vi "Get Message Fields.vi"(8 "error in (no error)":errorcluster, 11 "Message ref in":u64) -> (0 "error out":errorcluster, 2 "Field refs":u64[](array[numeric]), 3 "Message ref out":u64)   [LabVIEW 2019, in "gRPC Scripting Tools.lvlib"]
uses:
  gRPC Scripting Tools.lvlib
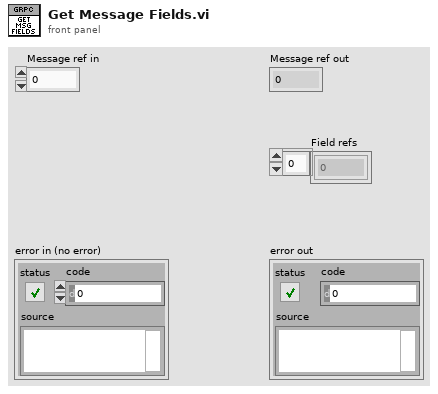
[diagram p1: front panel]
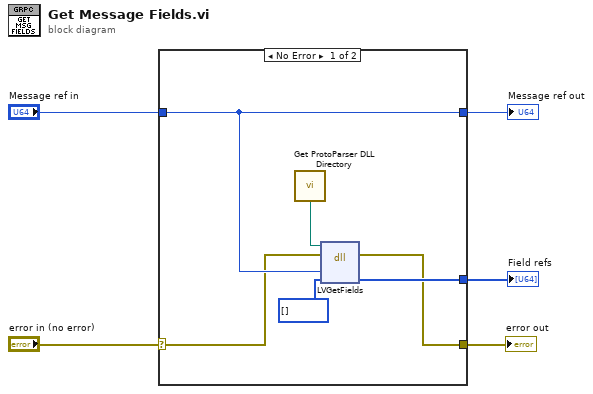
[diagram p0: block diagram]
diagram:
  n1 = case shown="No Error" "error in (no error)" {
    selector: "error in (no error)" -> [w7 w12]
    tunnel: "Message ref in" -> [w8 w13]
    tunnel: [w10 _] -> w4
    tunnel: [w8 w13] -> w3
    tunnel: [w6 w12] -> w1
    frame No Error {
      n2 = call "Get ProtoParser DLL Directory.vi"() -> ("Proto Parser Directory"=w9:path)
      n3 = dll-call lib="C:/Users/XEnderMD/Desktop/LV gRPC/labview source/gRPC Scripting Tools/Proto Parser API/dll/labview_grpc_generator.dll" fn="LVGetFields"(path in=w9, error in=w7, "message"=w8, "fieldInfo"=u64[] []) -> (error out=w6:errorcluster, "fieldInfo"=w10:u64[])  [unwired: 3 in, 1 out]
    }
    frame Error {
    }
  }
  "Field refs" <- w4
  "Message ref out" <- w3
  "error out" <- w1
